vi "Create Data Server Thread.vi"(8 "error in (no error)":errorcluster, 11 "Plugins":refnum<class "Plugin.lvclass">[](array[class])) -> (0 "error out":errorcluster, 3 "Data Server Thread out":refnum<class "Data Server Thread.lvclass">)   [LabVIEW 2017, in "DSF Core.lvlib" / "Data Server Thread.lvclass"]
uses:
  Data Server Thread.lvclass
  Plugin/Plugin.lvclass
  Data Server Thread.lvclass/Data Server Thread.ctl
  Buffer Map/Buffers Map.lvclass
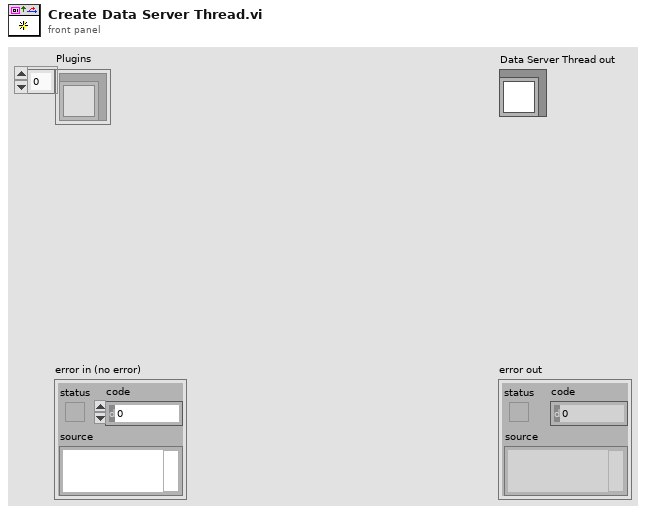
[diagram p1: front panel]
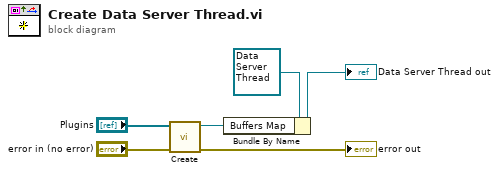
[diagram p0: block diagram]
diagram:
  n1 = call "Create.vi"("error in (no error)"="error in (no error)", "Plugins"="Plugins") -> ("error out"=→"error out":errorcluster, "Buffers Map out"=w6:refnum<class "Buffers Map.lvclass">)  [unwired: 8 in]
  n2 = Bundle By Name(cluster=refnum<class "Data Server Thread.lvclass"> refnum ("Data Server Thread out"), "Buffers Map"=w6) -> (→"Data Server Thread out":refnum<class "Data Server Thread.lvclass">)
